vi "Set value by Variant.vi"(8 "error in (no error)":errorcluster, 10 "Variant":variant, 11 "Text Column in":refnum<class "String Column.lvclass">) -> (0 "error out":errorcluster, 3 "Text Column out":refnum<class "String Column.lvclass">)   [LabVIEW 2020, in "Basic Columns.lvlib" / "String Column.lvclass"]
uses:
  String Column.lvclass
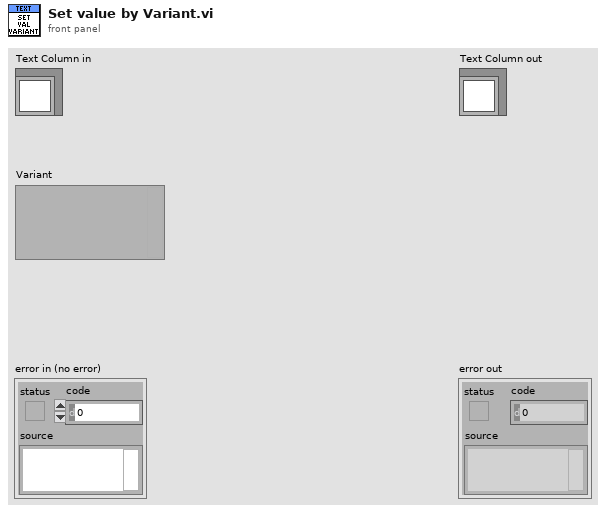
[diagram p1: front panel]
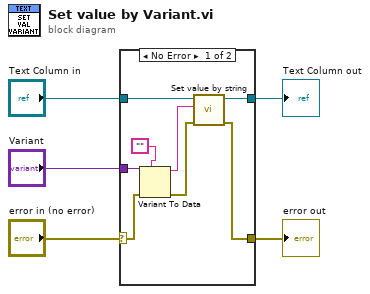
[diagram p0: block diagram]
diagram:
  n1 = case shown="No Error" "error in (no error)" {
    selector: "error in (no error)" -> [w12 w14]
    tunnel: [w7 w14] -> w4
    tunnel: "Text Column in" -> [w10 w15]
    tunnel: [w9 w15] -> w2
    tunnel: "Variant" -> [w13 _]
    frame No Error {
      n2 = Variant To Data(error in=w12, type="", Variant=w13) -> (data=w6:string, error out=w8:errorcluster)
      n3 = call-dynamic "Set value by string.vi"("error in (no error)"=w8, "Value"=w6, "Column in"=w10) -> ("error out"=w7:errorcluster, "Column out"=w9:refnum<class "String Column.lvclass">)  [unwired: 7 in]
    }
    frame Error {
    }
  }
  "error out" <- w4
  "Text Column out" <- w2
